vi "save_infos2.vi"() -> ()   [LabVIEW 2013]
panel:
  in  "Version":string="f"
  in  "Camera Serial":string="f"
  in  "Camera Model":string="f"
  in  "SOFT_VERSION":string="V2"
  in  "info Directory":path=path "D:/CONFIGS_TIME_LAPSE"
  in  "USED_FILTERS":u8[](array[numeric])
  in  "USED_LEDS":bool[][](array[boolean])=[[FALSE, FALSE], [TRUE, TRUE]]
  in  "Nstart":u32=30 step=1
  in  "Non":u32=150 step=1
  in  "Noff":u32 step=1
  in  "BETWEEN_PAT":u32
  in  "NPAT":u32
  in  "BETWEEN_SCAN":u32
  in  "NSCAN":u32
  in  "STAGE_PORT":refnum<visa-resource-name>="COM1"
  in  "STAGE_SPEED":dbl
  in  "ROMODE":u32
  in  "BIN":u16
  in  "EXPT":dbl
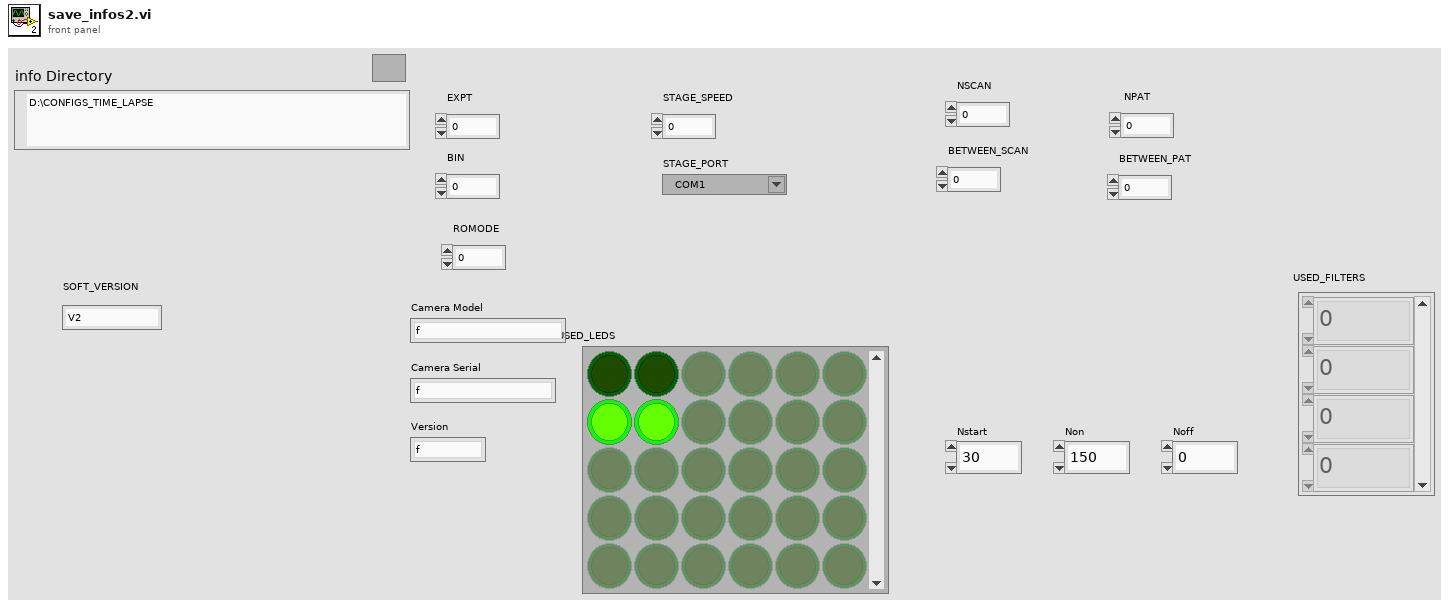
[diagram p1: front panel]
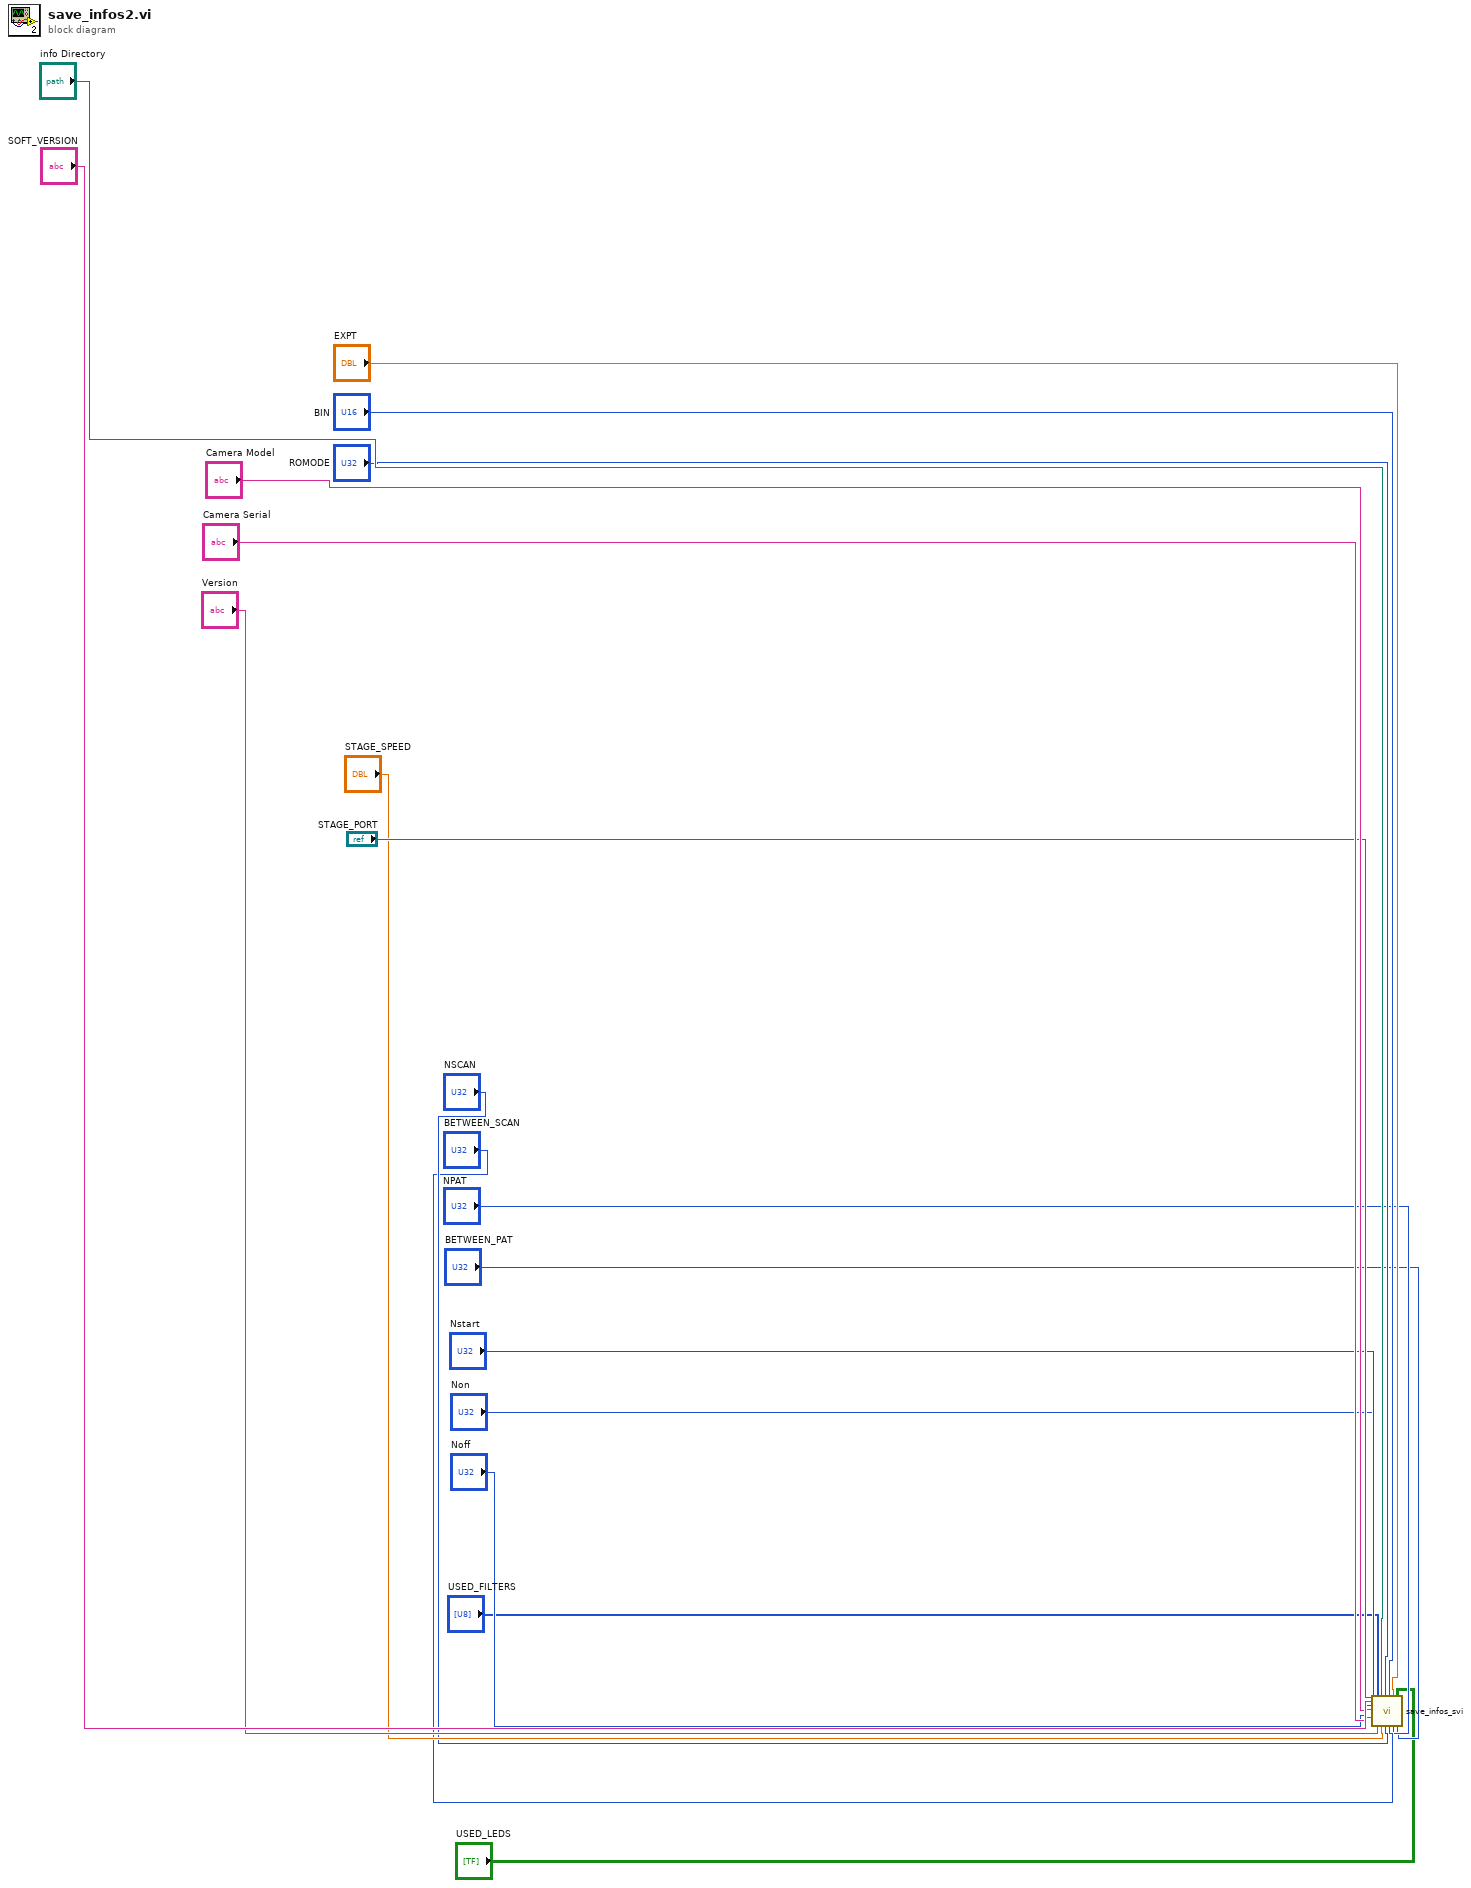
[diagram p0: block diagram]
diagram:
  n1 = call "save_infos_svi.vi"("Refnum VISA en entrée"="STAGE_PORT", "SOFT_VERSION"="SOFT_VERSION", "Noff"="Noff", "Camera Model"="Camera Model", "Non"="Non", "Camera Serial"="Camera Serial", "Nstart"="Nstart", "USED_FILTERS"="USED_FILTERS", "Version"="Version", "info Directory"="info Directory", "STAGE_SPEED"="STAGE_SPEED", "ROMODE"="ROMODE", "NSCAN"="NSCAN", "BIN"="BIN", "BETWEEN_SCAN"="BETWEEN_SCAN", "EXPT"="EXPT", "NPAT"="NPAT", "USED_LEDS"="USED_LEDS", "BETWEEN_PAT"="BETWEEN_PAT") -> ()  [unwired: 9 in]
